vi "Convert CAN Frame to RAW Frame.vi"(4 "CAN frame":T1={"timestamp"=timestamp(0 s since 1904-01-01), "payload"=[0, 0, 0, 0, 0, 0, 0, 0], "identifier"=0, "type"=0, "extended?"=FALSE, "echo?"=FALSE} {"payload" format="%x"; "timestamp" format="%<%.7X\n%x>T"; "type" items=["CAN Data"=0, "CAN Remote"=1, "CAN Bus Error"=2, "J1939 Data"=192, "Delay"=224, "Log Trigger"=225, "Start Trigger"=226]; "identifier" format="%x"}) -> (1 "RAW Data":u8[](array[numeric]) format="%.0x")   [LabVIEW 2013, in "J1939.lvlib"]
uses:
  J1939.lvlib
  <vilib>/xnet/xnet.llb/XNET Frame CAN.ctl
  <vilib>/xnet/xnet.llb/XNET Frame Type CAN.ctl
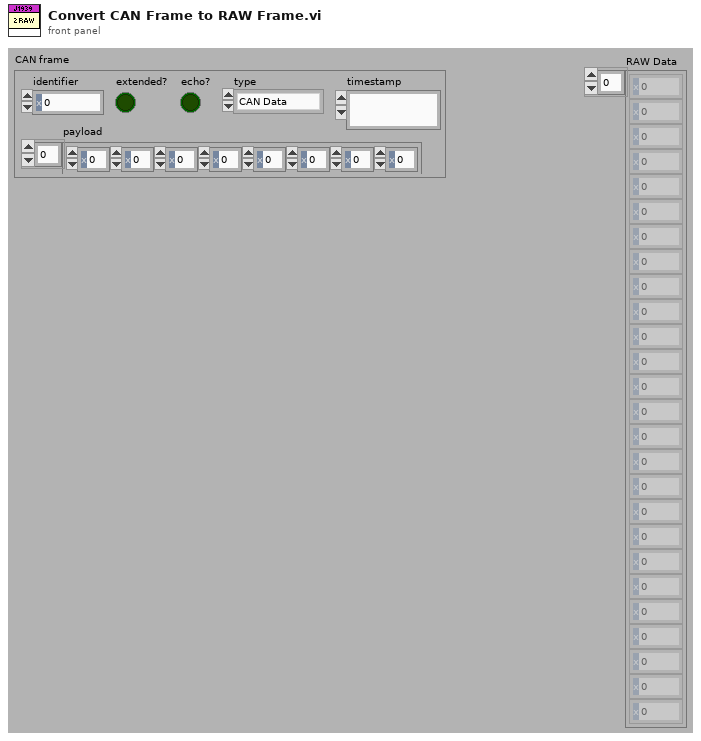
[diagram p1: front panel]
types:
  T1 = typedef "XNET Frame CAN.ctl" = cluster{"timestamp":timestamp, "payload":u8[], "identifier":u32, "type":T2, "extended?":bool, "echo?":bool}
  T2 = typedef "XNET Frame Type CAN.ctl" = u8
  T3 = enum16{"big-endian, network order", "native, host order", "little-endian"}
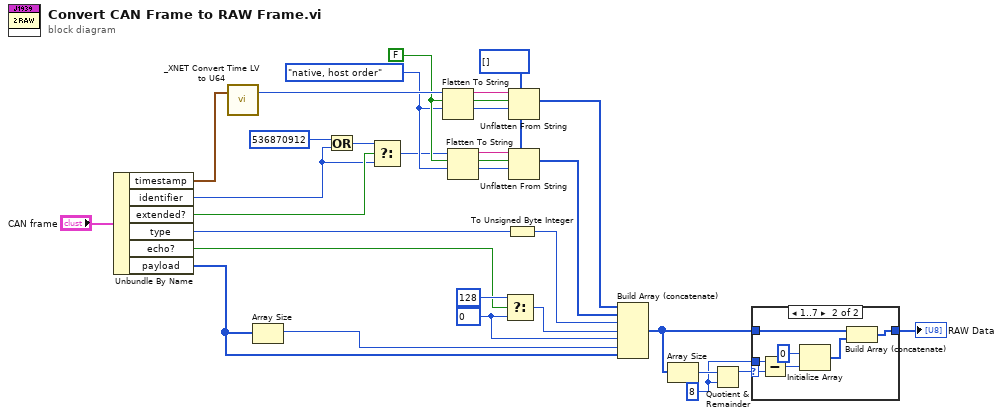
[diagram p0: block diagram]
diagram:
  w5 = 8 ("y")
  w10 = u8 0
  w7 = u8[] [] ("subarray")
  w23 = FALSE ("prepend array or string size? (T)")
  w22 = T3."native, host order" ("byte order (0:big-endian, network order)")
  n1 = Unbundle By Name("CAN frame") -> ("timestamp"=w28:timestamp, "identifier"=w17:u32, "extended?"=w19:bool, "type"=w8:T2, "echo?"=w14:bool, "payload"=w11:u8[])
  n2 = call <vilib>:"_XNET Convert Time LV to U64.vi"("Time LV"=w28) -> ("Time U64"=w27:u64)  [unwired: 2 in]
  n3 = Array Size(array=w11) -> (size(s)=w9:i32)
  n4 = Or(x=u32 536870912, y=w17) -> (x .or. y?=w18:u32)
  n5 = Select(t=w18, s=w19, f=w17) -> (s? t:f=w16:u32)
  n6 = Flatten To String(anything=w27, prepend array or string size? (T)=w23, byte order (0:big-endian, network order)=w22) -> (data string=w26:string)  [unwired: 1 in, 2 out]
  n7 = Flatten To String(anything=w16, prepend array or string size? (T)=w23, byte order (0:big-endian, network order)=w22) -> (data string=w24:string)  [unwired: 1 in, 2 out]
  n8 = Select(t=u8 128, s=w14, f=w10) -> (s? t:f=w13:u8)
  n9 = To Unsigned Byte Integer(number=w8) -> (unsigned 8bit integer=w12:T2)
  n10 = Unflatten From String(type=w7, binary string=w26, data includes array or string size? (T)=w23, byte order (0:big-endian, network order)=w22) -> (value=w25:u8[])  [unwired: 1 in, 2 out]
  n11 = Unflatten From String(type=w7, binary string=w24, data includes array or string size? (T)=w23, byte order (0:big-endian, network order)=w22) -> (value=w21:u8[])  [unwired: 1 in, 2 out]
  n12 = Build Array (concatenate)(w25, w21, w12, w13, w10, w9, w11) -> (w3:i32[])
  n13 = Array Size(array=w3) -> (size(s)=w6:i32)
  n14 = Quotient & Remainder(x=w6, y=w5) -> (x-y*floor(x/y)=w4:i32)  [unwired: 1 out]
  n15 = case shown="1..7" w4 {
    selector: w4 -> [_ w30]
    tunnel: w5 -> [_ w36]
    tunnel: w3 -> [w29 w32]
    tunnel: [w29 w31] -> w2
    frame 0, Default {
    }
    frame 1..7 {
      n16 = Subtract(x=w36, y=w30) -> (x-y=w35:i32)
      n17 = Initialize Array(u8 0 ("Numeric"), w35) -> (w33:u8[])
      n18 = Build Array (concatenate)(w32, w33) -> (w31:i32[])
    }
  }
  "RAW Data" <- w2
